vi "Assign Point Ramping.vi"(0 "Accurus Ctrl Cluster":T1={"Stop Accurus"=TRUE, "Vacuum Force"=0, "Max Limit [mmHg]"=600.0, "Slide in"=0} {"Slide in" scale=0.0..78.0; "Vacuum Force" min=0 max=78}, 4 "stop":bool, 5 "Ramp Time [sec]":dbl=3.0, 6 "L1 to L4 PID Cluster":T2={"L1 PID Gains"={"Kp"=0.005, "Kd"=0.5, "Ki"=0.0005}, "L2 PID Gains"={"Kp"=0.01, "Kd"=1.0, "Ki"=0.0005}, "L3 PID Gains"={"Kp"=0.05, "Kd"=1.0, "Ki"=0.0005}, "L4 PID Gains"={"Kp"=0.1, "Kd"=0.1, "Ki"=0.0005}}, 7 "Offset Home2RCM":dbl[](array[numeric])=[0.0, 0.0, 0.0, 0.0], 8 "Destination Posit Array [mm]":dbl[](array[numeric])=[0.0, 0.0, -3.0, 0.0], 9 "Previous Posit Array":dbl[](array[numeric])=[0.0, 0.0, 0.0, 0.0], 10 "error in":errorcluster, 11 "FPGA VI Reference In":refnum<k20>) -> (1 "Last L1 to L4 Posit":dbl[](array[numeric]), 2 "error out":errorcluster, 3 "FPGA VI Reference Out":refnum<k20>)   [LabVIEW 2016]
uses:
  <vilib>/Analysis/1siggen.llb/Ramp Pattern by Samples.vi
  Subsystems/Global Variables v1.vi
  <vilib>/Analysis/NI_AALBase.lvlib
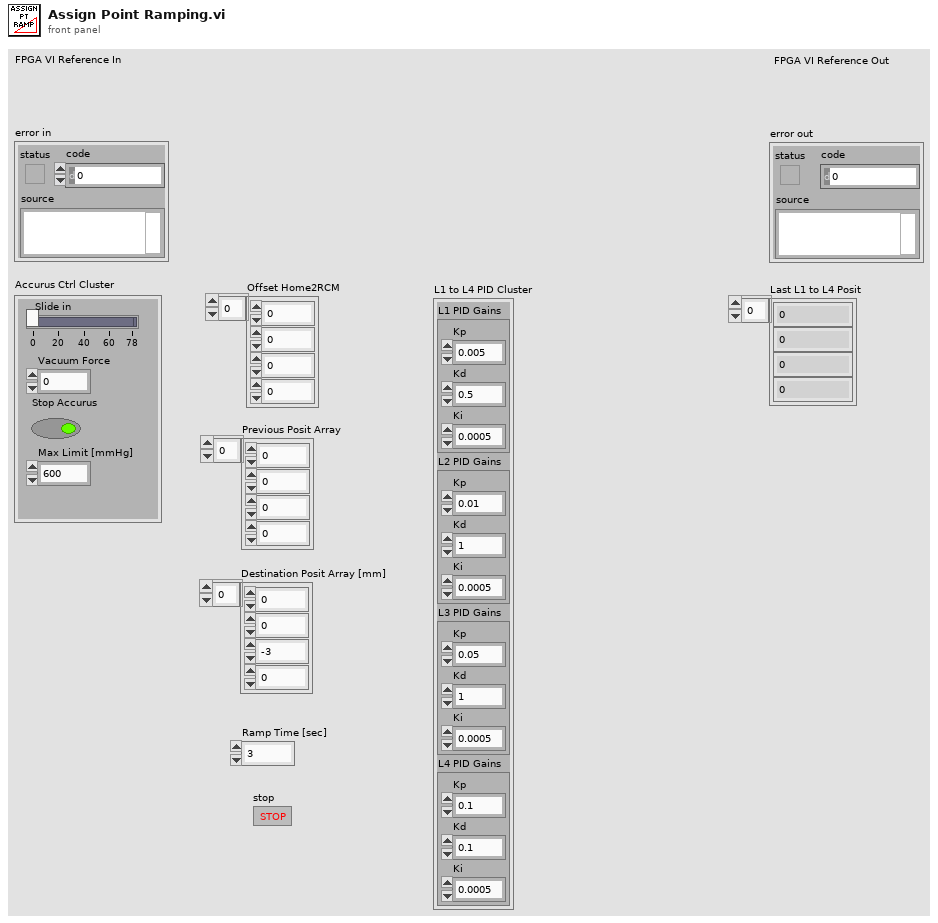
[diagram p1: front panel]
types:
  T1 = cluster{"Stop Accurus":bool, "Vacuum Force":i8, "Max Limit [mmHg]":dbl, "Slide in":i8}
  T2 = cluster{"L1 PID Gains":cluster{"Kp":dbl, "Kd":dbl, "Ki":dbl}, "L2 PID Gains":cluster{"Kp":dbl, "Kd":dbl, "Ki":dbl}, "L3 PID Gains":cluster{"Kp":dbl, "Kd":dbl, "Ki":dbl}, "L4 PID Gains":cluster{"Kp":dbl, "Kd":dbl, "Ki":dbl}}
  T3 = cluster{"Accurus button":bool[], "Vacuum engaged?":bool, "Vacuum Force":i32, "Accurus Ch. A Vout":dbl, "Accurus Ch. B Vout":dbl}
  T4 = cluster{"Vacuum Engaged?":bool, "Voltage Ouptut Ch. A":dbl, "Voltage Ouptut Ch. B":dbl, "Vacuum Force [mmHg]":i32, "Foot Paddle 3":dbl}
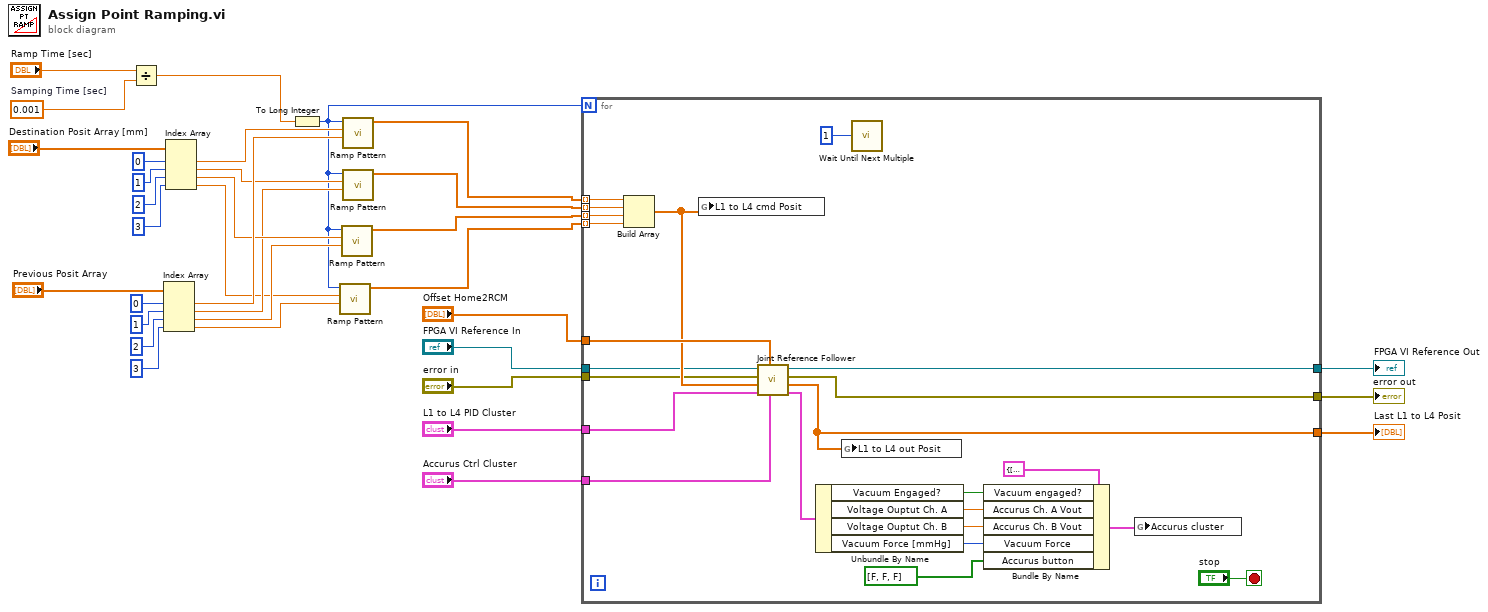
[diagram p0: block diagram]
diagram:
  w23 = 0.001  # Samping Time [sec]
  n1 = Divide(x="Ramp Time [sec]", y=w23) -> (x/y=w14:dbl)
  n2 = Index Array(array="Previous Posit Array", index #1=0 ("index"), index #2=1 ("index"), index #3=2 ("index"), index #4=3 ("index")) -> (element #1=w22:dbl, element #2=w18:dbl, element #3=w17:dbl, element #4=w16:dbl)
  n3 = Index Array(array="Destination Posit Array [mm]", index #1=0 ("index"), index #2=1 ("index"), index #3=2 ("index"), index #4=3 ("index")) -> (element #1=w21:dbl, element #2=w20:dbl, element #3=w19:dbl, element #4=w15:dbl)
  n4 = To Long Integer(number=w14) -> (32bit integer=w13:i32)
  n5 = call-poly <vilib>:"Ramp Pattern.vi"("start"=w16, "end"=w15, "samples"=w13) -> ("Ramp Pattern"=w9:dbl[])  [unwired: 7 in, 1 out]
  n6 = call-poly <vilib>:"Ramp Pattern.vi"("start"=w17, "end"=w19, "samples"=w13) -> ("Ramp Pattern"=w10:dbl[])  [unwired: 7 in, 1 out]
  n7 = call-poly <vilib>:"Ramp Pattern.vi"("start"=w22, "end"=w21, "samples"=w13) -> ("Ramp Pattern"=w12:dbl[])  [unwired: 7 in, 1 out]
  n8 = call-poly <vilib>:"Ramp Pattern.vi"("start"=w18, "end"=w20, "samples"=w13) -> ("Ramp Pattern"=w11:dbl[])  [unwired: 7 in, 1 out]
  n9 = for {
    N: w13 -> [_]
    tunnel: w12 -> [w57] mode=indexing
    tunnel: w11 -> [w56] mode=indexing
    tunnel: w10 -> [w55] mode=indexing
    tunnel: w9 -> [w54] mode=indexing
    tunnel: [w52] -> w5
    tunnel: [w51] -> w4
    tunnel: "Offset Home2RCM" -> [w50]
    tunnel: "L1 to L4 PID Cluster" -> [w49]
    tunnel: [w47] -> w7
    tunnel: "FPGA VI Reference In" -> [w45]
    tunnel: "error in" -> [w44]
    tunnel: "Accurus Ctrl Cluster" -> [w35]
    stop <- "stop" stop-if-true
    n10 = Build Array(w57, w56, w55, w54) -> (w48:dbl[])
    n11 = global write "Global Variables v1.vi" "L1 to L4 cmd Posit"(w48) -> ()
    n12 = call "Joint Reference Follower.vi"("Accurus Ctrl Cluster"=w35, "Offset Home2RCM [deg/mm]"=w50, "PID Ctrl Cluster"=w49, "Ref Array [deg/mm]"=w48, "error in"=w44, "FPGA VI Reference In"=w45) -> ("Accurus Output Cluster"=w37:T4, "Output Posit Array [deg/mm]"=w47:dbl[], "error out"=w51:errorcluster, "FPGA VI Reference Out"=w52:refnum<k20>)  [unwired: 2 in]
    n13 = Unbundle By Name(w37) -> ("Vacuum Engaged?"=w42:bool, "Voltage Ouptut Ch. A"=w41:dbl, "Voltage Ouptut Ch. B"=w40:dbl, "Vacuum Force [mmHg]"=w39:i32)
    n14 = global write "Global Variables v1.vi" "L1 to L4 out Posit"(w47) -> ()
    n15 = call "Wait Until Next Multiple"("Count(mSec)"=u32 1) -> ()  [unwired: 1 out]
    n16 = Bundle By Name(cluster=T3 {"Accurus button"=[TRUE, TRUE, TRUE], "Vacuum engaged?"=TRUE, "Vacuum Force"=0, "Accurus Ch. A Vout"=0.0, "Accurus Ch. B Vout"=0.0} ("Accurus cluster"), "Vacuum engaged?"=w42, "Accurus Ch. A Vout"=w41, "Accurus Ch. B Vout"=w40, "Vacuum Force"=w39, "Accurus button"=bool[] [FALSE, FALSE, FALSE]) -> (w43:T3)
    n17 = global write "Global Variables v1.vi" "Accurus cluster"(w43) -> ()
  }
  "error out" <- w4
  "FPGA VI Reference Out" <- w5
  "Last L1 to L4 Posit" <- w7
